vi "StaticSetPoint.vi"(0 "COMPORT":refnum<visa-resource-name>="COM1", 5 "ILabVIEW":refnum<k24>, 7 "Set Point":dbl format="%.3g", 11 "Error In":errorcluster, 12 "R(t)":bool, 13 "close session(t)":bool=TRUE, 14 "W(t)":bool) -> (3 "x = y?":bool, 4 "comport":refnum<visa-resource-name>="COM1", 6 "ILabVIEW Out":refnum<k24>, 15 "error out":errorcluster)   [LabVIEW 2018]
uses:
  C:/RageATE/Instruments/Ess Temp Plate/LabView Driver/Public/Watbus.dll
  LabView Driver/Public/Watbus.dll
panel:
  in  "OpenSession(t)":bool
  in  "TemperatureUnits":u8(ring)=1 items=["Degrees F", "Degrees C"]
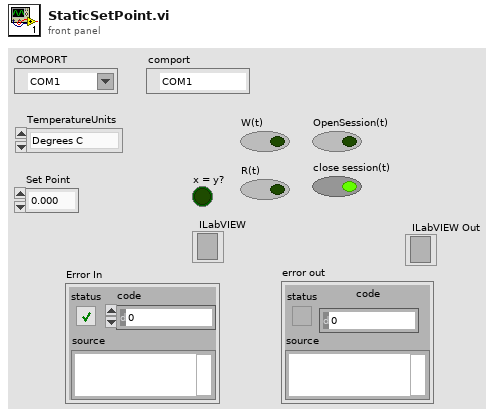
[diagram p1: front panel]
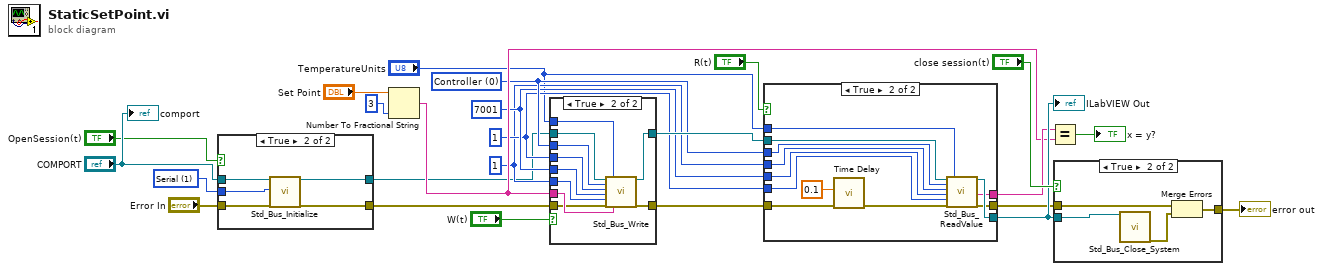
[diagram p0: block diagram]
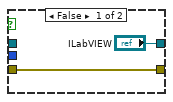
[diagram p2: hidden frame]
diagram:
  w10 = 1 items=["Usb", "Serial", "Ethernet", "Unconnected"] ("InterfaceType")
  w17 = 0 items=["Controller", "RUI", "PC", "CommsCard"] ("deviceType")
  w14 = 1 ("InstanceId")
  w15 = 1 ("Zone")
  w16 = 7001 ("ParameterID")
  n1 = case shown="True" "OpenSession(t)" {
    tunnel: "COMPORT" -> [_ w31]
    tunnel: w10 -> [_ w30]
    tunnel: "Error In" -> [w25 w29]
    tunnel: [w25 w28] -> w1
    tunnel: ["ILabVIEW" w27] -> w9
    frame False {
    }
    frame True {
      n2 = call "Std_Bus_Initialize.vi"("Communications Port"=w31, "InterfaceType"=w30, "error in (no error)"=w29) -> ("ILabVIEW"=w27:refnum<k24>, "error out"=w28:errorcluster)  [unwired: 14 in, 1 out]
    }
  }
  n3 = Number To Fractional String(number="Set Point", precision (6)=i16 3) -> (F-format string=w18:string)  [unwired: 2 in]
  n4 = case shown="True" "W(t)" {
    tunnel: [w32 w43] -> w22
    tunnel: [w33 w42] -> w21
    tunnel: w18 -> [_ w41]
    tunnel: "TemperatureUnits" -> [_ w40]
    tunnel: w17 -> [_ w39]
    tunnel: w16 -> [_ w38]
    tunnel: w15 -> [_ w37]
    tunnel: w14 -> [_ w36]
    tunnel: w1 -> [w33 w35]
    tunnel: w9 -> [w32 w34]
    frame False {
    }
    frame True {
      n5 = call "Std_Bus_Write.vi"("ILabVIEW In"=w34, "deviceType"=w39, "Zone"=w37, "ParameterID"=w38, "InstanceId"=w36, "error in (no error)"=w35, "TemperatureUnits"=w40, "WriteValue"=w41) -> ("ILabVIEW Out"=w43:refnum<k24>, "error out"=w42:errorcluster)  [unwired: 10 in]
    }
  }
  n6 = case shown="True" "R(t)" {
    tunnel: w22 -> [w45 w57]
    tunnel: w21 -> [w44 w56]
    tunnel: [w45 w55] -> w20
    tunnel: [_ w54] -> w19
    tunnel: "TemperatureUnits" -> [_ w53]
    tunnel: w17 -> [_ w52]
    tunnel: w16 -> [_ w51]
    tunnel: w15 -> [_ w50]
    tunnel: w14 -> [_ w49]
    tunnel: [w44 w46] -> w4
    frame False {
    }
    frame True {
      n7 = call "Time Delay"("error in (no error)"=w56, "Delay Time (s)"=0.1) -> ("error out"=w48:errorcluster)  [unwired: 9 in]
      n8 = call "Std_Bus_ReadValue.vi"("ILabVIEW In"=w57, "DeviceType"=w52, "Zone"=w49, "ParameterID"=w51, "InstanceId"=w50, "error in (no error)"=w48, "TemperatureUnits"=w53) -> ("ILabVIEW Out"=w55:refnum<k24>, "Value Out"=w54:string, "error out"=w46:errorcluster)  [unwired: 10 in]
    }
  }
  "ILabVIEW Out" <- w20
  n9 = Equal?(x=w19, y=w18) -> (x = y?=→"x = y?":bool)
  n10 = case shown="True" "close session(t)" {
    tunnel: w20 -> [_ w62]
    tunnel: [w58 w59] -> w5
    tunnel: w4 -> [w58 w61]
    frame False {
    }
    frame True {
      n11 = call "Std_Bus_Close_System.vi"("ILabVIEW In"=w62) -> ("error out"=w60:errorcluster)  [unwired: 18 in]
      n12 = Merge Errors(w61, w60) -> (w59:errorcluster)
    }
  }
  "error out" <- w5
  "comport" <- "COMPORT"
